vi "NI 9260 Synchronization 9775 (Host).vi"() -> ()   [LabVIEW 2021]
uses:
  <vilib>/LabVIEW Targets/FPGA/cRIO/shared/nicrio_ModuleControls/nicrio_cRIO-9260_DataRatesRing2.ctl
  <vilib>/LabVIEW Targets/FPGA/cRIO/shared/nicrio_ModuleControls/nicrio_cRIO-9775_RecordDataRates4ChansRing.ctl
  <vilib>/FPGAPlugInAG/cRIO-9053/niLvFpga_Open_cRIO-9053.vi
  <vilib>/rvi/interface/common/dynamic/niFpgaDynamicAddResources.vi
  <vilib>/Utility/error.llb/Error Cluster From Error Code.vi
  <vilib>/rvi/errors/niLvFpgaAdjustHostInterfaceError.vi
  <vilib>/rvi/interface/common/niFpgaWaitOnOcc.vi
  <vilib>/FPGAPlugInAG/Dynamic/niLvFpga_Run_Dynamic.vi
  <vilib>/FPGAPlugInAG/Dynamic/niLvFpga_Close_Dynamic.vi
  <vilib>/rvi/interface/nirviOpenFPGA/nirviOpenFPGA.xnode
  FPGA Bitfiles/crio-ni9260_FPGATarget_NI9260Synchroniz_lbmddMo-IB0.lvbitx
  NI 9260 Synchronization 9775 (FPGA).vi
  <vilib>/rvi/interface/nirviReadWriteControl/nirviReadWriteControl.xnode
  <vilib>/rvi/interface/nirviMethod/nirviMethod.xnode
  <vilib>/rvi/interface/nirviCloseFPGA/nirviCloseFPGA.xnode
  <vilib>/rvi/interface/Simulation/niFpgaSimulationCallBeginRW.vi
  <vilib>/FPGAPlugInAG/Dynamic/niLvFpga_WriteFifo_Dynamic.vi
  <vilib>/rvi/errors/niLvFpgaMergeErrorWithErrorCode.vi
  <vilib>/FPGAPlugInAG/Dynamic/niLvFpga_ConfigureFifo_Dynamic.vi
  <vilib>/Analysis/NI_AALPro.lvlib
  NiFpgaLv.dll
  <vilib>/FPGAPlugInAG/Dynamic/niLvFpga_ReadFifo_Dynamic.vi
panel:
  in  "NI9775 Data Rate":T1=1 items=["20.000 MS/s (NI 9775)"=1, "10.00 MS/s (NI 9775)"=2, "6.667 MS/s (NI 9775)"=3, "5.000 MS/s (NI 9775)"=4, "2.500 MS/s (NI 9775)"=8, "1.667 MS/s (NI 9775)"=12, "1.250 MS/s (NI 9775)"=16, "1.000 MS/s (NI 9775)"=20, "833.333 KS/s (NI 9775)"=24, "714.286 KS/s (NI 9775)"=28, "625.000 KS/s (NI 9775)"=32, "555.556 KS/s (NI 9775)"=36, "500.000 KS/s (NI 9775)"=40, "454.545 KS/s (NI 9775)"=44, "416.667 KS/s (NI 9775)"=48, "384.615 KS/s (NI 9775)"=52, "357.143 KS/s (NI 9775)"=56, "333.333 KS/s (NI 9775)"=60, "312.500 KS/s (NI 9775)"=64, "294.118 KS/s (NI 9775)"=68, "277.778 KS/s (NI 9775)"=72, "263.158 KS/s (NI 9775)"=76, "250.000 KS/s (NI 9775)"=80, "238.095 KS/s (NI 9775)"=84, "227.273 KS/s (NI 9775)"=88, "217.391 KS/s (NI 9775)"=92, "208.333 KS/s (NI 9775)"=96, "200.000 KS/s (NI 9775)"=100, "192.308 KS/s (NI 9775)"=104, "185.185 KS/s (NI 9775)"=108, "178.571 KS/s (NI 9775)"=112, "172.414 KS/s (NI 9775)"=116, "166.667 KS/s (NI 9775)"=120, "161.290 KS/s (NI 9775)"=124, "156.250 KS/s (NI 9775)"=128, "151.515 KS/s (NI 9775)"=132, "147.059 KS/s (NI 9775)"=136, "142.857 KS/s (NI 9775)"=140, "138.889 KS/s (NI 9775)"=144, "135.135 KS/s (NI 9775)"=148, "131.579 KS/s (NI 9775)"=152, "128.205 KS/s (NI 9775)"=156, "125.000 KS/s (NI 9775)"=160, "121.951 KS/s (NI 9775)"=164, "119.048 KS/s (NI 9775)"=168, "116.279 KS/s (NI 9775)"=172, "113.636 KS/s (NI 9775)"=176, "111.111 KS/s (NI 9775)"=180, "108.696 KS/s (NI 9775)"=184, "106.383 KS/s (NI 9775)"=188, "104.167 KS/s (NI 9775)"=192, "102.041 KS/s (NI 9775)"=196, "100.000 KS/s (NI 9775)"=200, "50.000 KS/s (NI 9775)"=400, "33.333 KS/s (NI 9775)"=600, "25.000 KS/s (NI 9775)"=800, "20.000 KS/s (NI 9775)"=1000, "16.667 KS/s (NI 9775)"=1200, "14.286 KS/s (NI 9775)"=1400, "12.500 KS/s (NI 9775)"=1600, "11.111 KS/s (NI 9775)"=1800, "10.000 KS/s (NI 9775)"=2000, "9.091 KS/s (NI 9775)"=2200, "8.333 KS/s (NI 9775)"=2400, "7.692 KS/s (NI 9775)"=2600, "7.143 KS/s (NI 9775)"=2800, "6.667 KS/s (NI 9775)"=3000, "6.250 KS/s (NI 9775)"=3200, "5.882 KS/s (NI 9775)"=3400, "5.556 KS/s (NI 9775)"=3600, "5.000 KS/s (NI 9775)"=4000, "4.762 KS/s (NI 9775)"=4200, "4.545 KS/s (NI 9775)"=4400, "4.348 KS/s (NI 9775)"=4600, "4.167 KS/s (NI 9775)"=4800, "4.000 KS/s (NI 9775)"=5000, "3.846 KS/s (NI 9775)"=5200, "3.571 KS/s (NI 9775)"=5600, "3.333 KS/s (NI 9775)"=6000, "3.125 KS/s (NI 9775)"=6400, "2.941 KS/s (NI 9775)"=6800, "2.778 KS/s (NI 9775)"=7200, "2.632 KS/s (NI 9775)"=7600, "2.500 KS/s (NI 9775)"=8000, "2.381 KS/s (NI 9775)"=8400, "2.273 KS/s (NI 9775)"=8800, "2.174 KS/s (NI 9775)"=9200, "2.083 KS/s (NI 9775)"=9600, "2.000 KS/s (NI 9775)"=10000, "1.923 KS/s (NI 9775)"=10400, "1.852 KS/s (NI 9775)"=10800, "1.786 KS/s (NI 9775)"=11200, "1.724 KS/s (NI 9775)"=11600, "1.667 KS/s (NI 9775)"=12000, "1.613 KS/s (NI 9775)"=12400, "1.563 KS/s (NI 9775)"=12800, "1.515 KS/s (NI 9775)"=13200, "1.471 KS/s (NI 9775)"=13600, "1.429 KS/s (NI 9775)"=14000, "1.389 KS/s (NI 9775)"=14400, "1.351 KS/s (NI 9775)"=14800, "1.316 KS/s (NI 9775)"=15200, "1.282 KS/s (NI 9775)"=15600, "1.250 KS/s (NI 9775)"=16000, "1.220 KS/s (NI 9775)"=16400, "1.190 KS/s (NI 9775)"=16800, "1.163 KS/s (NI 9775)"=17200, "1.136 KS/s (NI 9775)"=17600, "1.111 KS/s (NI 9775)"=18000, "1.087 KS/s (NI 9775)"=18400, "1.064 KS/s (NI 9775)"=18800, "1.042 KS/s (NI 9775)"=19200, "1.020 KS/s (NI 9775)"=19600, "1.000 KS/s (NI 9775)"=20000, "0.980 KS/s (NI 9775)"=20400, "0.962 KS/s (NI 9775)"=20800, "0.943 KS/s (NI 9775)"=21200, "0.926 KS/s (NI 9775)"=21600, "0.909 KS/s (NI 9775)"=22000, "0.893 KS/s (NI 9775)"=22400, "0.877 KS/s (NI 9775)"=22800, "0.862 KS/s (NI 9775)"=23200, "0.847 KS/s (NI 9775)"=23600, "0.833 KS/s (NI 9775)"=24000, "0.820 KS/s (NI 9775)"=24400, "0.806 KS/s (NI 9775)"=24800, "0.794 KS/s (NI 9775)"=25200, "0.781 KS/s (NI 9775)"=25600, "0.694 KS/s (NI 9775)"=28800, "0.625 KS/s (NI 9775)"=32000, "0.568 KS/s (NI 9775)"=35200, "0.521 KS/s (NI 9775)"=38400, "0.446 KS/s (NI 9775)"=44800, "0.391 KS/s (NI 9775)"=51200, "0.347 KS/s (NI 9775)"=57600, "0.313 KS/s (NI 9775)"=64000]
  out "host rate (ms)":u32
  out "Analog Input 2":waveform(dbl)(graph)
  in  "Waveform":T2(ring)=enum."Sine Wave"
  in  "NI 9260 Data Rate":T3=1 items=["51.200 kS/s (NI 9260)"=1, "25.600 kS/s (NI 9260)"=2, "17.067 kS/s (NI 9260)"=3, "12.800 kS/s (NI 9260)"=4, "10.240 kS/s (NI 9260)"=5, "8.533 kS/s (NI 9260)"=6, "7.314 kS/s (NI 9260)"=7, "6.400 kS/s (NI 9260)"=8, "5.689 kS/s (NI 9260)"=9, "5.120 kS/s (NI 9260)"=10, "4.654 kS/s (NI 9260)"=11, "4.267 kS/s (NI 9260)"=12, "3.938 kS/s (NI 9260)"=13, "3.657 kS/s (NI 9260)"=14, "3.413 kS/s (NI 9260)"=15, "3.200 kS/s (NI 9260)"=16, "3.012 kS/s (NI 9260)"=17, "2.845 kS/s (NI 9260)"=18, "2.695 kS/s (NI 9260)"=19, "2.560 kS/s (NI 9260)"=20, "2.438 kS/s (NI 9260)"=21, "2.328 kS/s (NI 9260)"=22, "2.226 kS/s (NI 9260)"=23, "2.133 kS/s (NI 9260)"=24, "2.048 kS/s (NI 9260)"=25, "1.969 kS/s (NI 9260)"=26, "1.896 kS/s (NI 9260)"=27, "1.829 kS/s (NI 9260)"=28, "1.765 kS/s (NI 9260)"=29, "1.707 kS/s (NI 9260)"=30, "1.652 kS/s (NI 9260)"=31]
  out "Analog Input":waveform(dbl)[](graph)
  out "NI 9230 FIFO Time Out":bool
  in  "Host Loop Rate (ms)":u32=100
  out "NI 9260 FIFO Time Out":bool
  in  "Waveform Settings":T4(array[cluster])=[{"Frequency (Hz)"=100.0, "Amplitude (V)"=3.0, "Offset (V)"=0.0, "Phase (deg)"=0.0}, {"Frequency (Hz)"=100.0, "Amplitude (V)"=3.0, "Offset (V)"=0.0, "Phase (deg)"=0.0}]
  in  "stop":bool
  out "FPGA Error out":errorcluster
  in  "Number of Samples per channel":dbl=2048.0 format="%.4p"
  out "Analog Output":waveform(dbl)[](graph)
  out "Host Error out":errorcluster
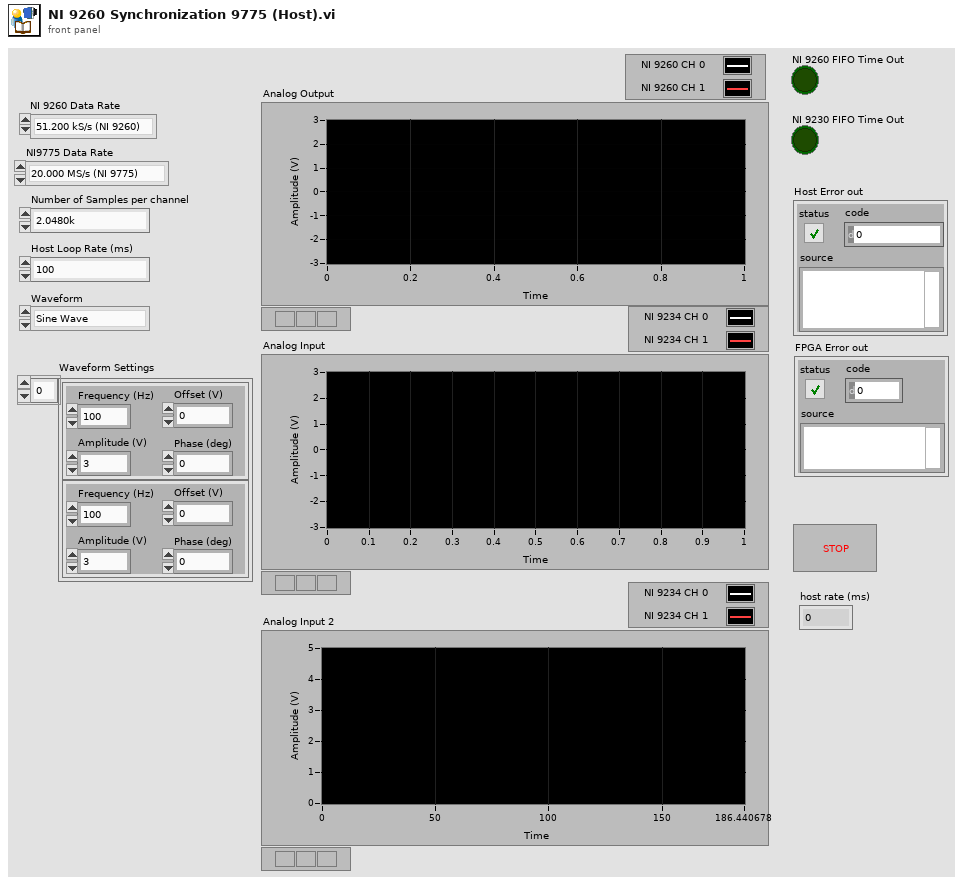
[diagram p1: front panel]
types:
  T1 = typedef "nicrio_cRIO-9775_RecordDataRates4ChansRing.ctl" = u16
  T2 = enum16{"Sawtooth Wave", "Square Wave", "Sine Wave"}
  T3 = typedef "nicrio_cRIO-9260_DataRatesRing2.ctl" = u8
  T4 = cluster{"Frequency (Hz)":dbl, "Amplitude (V)":dbl, "Offset (V)":dbl, "Phase (deg)":dbl}[]
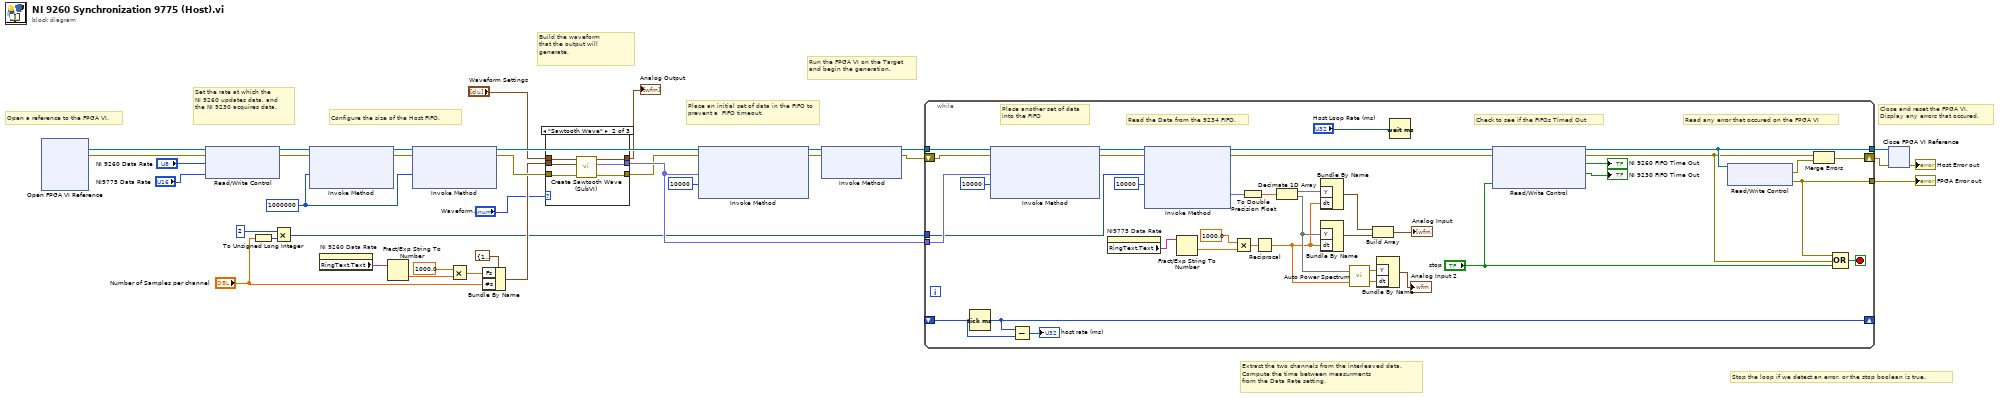
[diagram p0: block diagram]
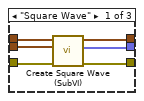
[diagram p2: hidden frame]
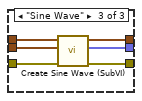
[diagram p3: hidden frame]
diagram:
  w2 = u32 1000000 ("Requested Depth")
  # "Build the waveform \nthat the output will generate."
  # "Extract the two channels from the interleaved data.\nCompute the time between measurments \nfrom the Data Rate setting."
  # "Place an initial set of data in the FIFO to prevent a  FIFO timeout."
  # "Stop the loop if we detect an error, or the stop boolean is true."
  # "Configure the size of the Host FIFO."
  # "Set the rate at which the \nNI 9260 updates data, and\nthe NI 9230 acquires data."
  # "Close and reset the FPGA VI. \nDisplay any errors that occured."
  # "Run the FPGA VI on the Target and begin the generation."
  # "Open a reference to the FPGA VI."
  n1 = xnode "Open FPGA VI Reference"() -> ("FPGA VI Reference Out"=w33:refnum<k20>, "error out"=w35:errorcluster)  [unwired: 2 in]
  n2 = xnode "Read/Write Control"("FPGA VI Reference In"=w33, "error in"=w35, "NI 9260 Data Rate"="NI 9260 Data Rate", "NI9775 Data Rate"="NI9775 Data Rate") -> ("FPGA VI Reference Out"=w15:refnum<k20>, "error out"=w23:errorcluster)
  n3 = To Unsigned Long Integer(number="Number of Samples per channel") -> (unsigned 32bit integer=w28:u32)
  n4 = Multiply(x=u32 2, y=w28) -> (x*y=w3:u32)
  n5 = xnode "Invoke Method"("FPGA VI Reference In"=w15, "error in"=w23, "Requested Depth"=w2) -> ("FPGA VI Reference Out"=w14:refnum<k20>, "error out"=w16:errorcluster)  [unwired: 1 out]
  n6 = property on="NI 9260 Data Rate" class="Ring (strict)"() -> ("RingText.Text"=w5:string)  [unwired: 2 in, 2 out]
  n7 = Fract/Exp String To Number(string=w5) -> (number=w31:dbl)  [unwired: 3 in, 1 out]
  n8 = xnode "Invoke Method"("FPGA VI Reference In"=w14, "error in"=w16, "Requested Depth"=w2) -> ("FPGA VI Reference Out"=w25:refnum<k20>, "error out"=w13:errorcluster)  [unwired: 1 out]
  n9 = Multiply(x=1000.0, y=w31) -> (x*y=w20:dbl)
  n10 = Bundle By Name(cluster=cluster{"Fs":dbl, "#s":dbl} {"Fs"=1000.0, "#s"=1000.0} ("sampling info"), "Fs"=w20, "#s"="Number of Samples per channel") -> (w11:cluster{"Fs":dbl, "#s":dbl})
  n11 = case shown="\"Sawtooth Wave\"" "Waveform" {
    tunnel: w13 -> [w39 w45 w53]
    tunnel: "Waveform Settings" -> [w41 w47 w52]
    tunnel: w11 -> [w40 w46 w51]
    tunnel: [w36 w42 w50] -> w10
    tunnel: [w38 w43 w49] -> w9
    tunnel: [w37 w44 w48] -> w7
    frame "Square Wave" {
      n12 = call "Create Square Wave (SubVI).vi"("error in (no error)"=w39, "sampling info"=w40, "Sine Waveform Settings"=w41) -> ("error out"=w38:errorcluster, "FXP Sinewave"=w36:fxp<+/-,24,4>[], "Voltage Output Waveform"=w37:waveform(dbl)[])  [unwired: 6 in]
    }
    frame "Sawtooth Wave" {
      n13 = call "Create Sawtooth Wave (SubVI).vi"("error in (no error)"=w45, "sampling info"=w46, "Sine Waveform Settings"=w47) -> ("error out"=w43:errorcluster, "FXP Sinewave"=w42:fxp<+/-,24,4>[], "Voltage Output Waveform"=w44:waveform(dbl)[])  [unwired: 6 in]
    }
    frame "Sine Wave" {
      n14 = call "Create Sine Wave (SubVI).vi"("error in (no error)"=w53, "sampling info"=w51, "Sine Waveform Settings"=w52) -> ("error out"=w49:errorcluster, "FXP Sinewave"=w50:fxp<+/-,24,4>[], "Voltage Output Waveform"=w48:waveform(dbl)[])  [unwired: 6 in]
    }
  }
  "Analog Output" <- w7
  n15 = xnode "Invoke Method"("FPGA VI Reference In"=w25, "error in"=w9, "Data"=w10, "Timeout (ms)"=10000) -> ("FPGA VI Reference Out"=w24:refnum<k20>, "error out"=w26:errorcluster)  [unwired: 1 out]
  n16 = xnode "Invoke Method"("FPGA VI Reference In"=w24, "error in"=w26) -> ("FPGA VI Reference Out"=w27:refnum<k20>, "error out"=w8:errorcluster)  [unwired: 1 in]
  n17 = while {
    tunnel: w27 -> [w91]
    tunnel: w10 -> [w90]
    tunnel: [w80] -> w21
    tunnel: [w86] -> w17
    shift-right: [w68] -> w30
    shift-left: w8 -> [w66]
    shift-right: [w58] -> _
    shift-left: _ -> [w57]
    tunnel: w3 -> [w55]
    stop <- w88 stop-if-true
    # "Check to see if the FIFOs Timed Out"
    # "Read any error that occured on the FPGA VI"
    # "Read the Data from the 9234 FIFO."
    # "Place another set of data\ninto the FIFO"
    n18 = Tick Count (ms)() -> (millisecond timer value=w58:u32)
    n19 = xnode "Invoke Method"("FPGA VI Reference In"=w91, "error in"=w66, "Data"=w90, "Timeout (ms)"=10000) -> ("FPGA VI Reference Out"=w85:refnum<k20>, "error out"=w84:errorcluster)  [unwired: 1 out]
    n20 = Subtract(x=w58, y=w57) -> (x-y=→"host rate (ms)":u32)
    n21 = property on="NI9775 Data Rate" class="Ring (strict)"() -> ("RingText.Text"=w54:string)  [unwired: 2 in, 2 out]
    n22 = xnode "Invoke Method"("FPGA VI Reference In"=w85, "error in"=w84, "Number of Elements"=w55, "Timeout (ms)"=10000) -> ("FPGA VI Reference Out"=w82:refnum<k20>, "error out"=w81:errorcluster, "Data"=w79:fxp<+/-,24,7>[])  [unwired: 1 out]
    n23 = Fract/Exp String To Number(string=w54) -> (number=w76:dbl)  [unwired: 4 out]
    n24 = Multiply(x=1000.0, y=w76) -> (x*y=w77:dbl)
    n25 = To Double Precision Float(number=w79) -> (double precision float=w69:dbl[])
    n26 = Reciprocal(x=w77) -> (1/x=w62:dbl)
    n27 = Decimate 1D Array(w69) -> (w73:dbl[], w63:dbl[])
    n28 = Bundle By Name("Y"=w73, "dt"=w62) -> (w75:waveform(dbl))  [unwired: 1 out]
    n29 = Bundle By Name("Y"=w63, "dt"=w62) -> (w74:waveform(dbl))  [unwired: 1 out]
    n30 = call <vilib>:"Auto Power Spectrum.vi"("dt"=w62, "Signal (V)"=w63) -> ("df"=w60:dbl, "Power Spectrum (V^2 rms)"=w61:dbl[])
    n31 = Build Array(w75, w74) -> (→"Analog Input":waveform(dbl)[])
    n32 = Bundle By Name("Y"=w61, "dt"=w60) -> (→"Analog Input 2":waveform(dbl))  [unwired: 1 out]
    n33 = Wait (ms)(milliseconds to wait="Host Loop Rate (ms)") -> ()  [unwired: 1 out]
    n34 = xnode "Read/Write Control"("FPGA VI Reference In"=w82, "error in"=w81, "stop"="stop") -> ("FPGA VI Reference Out"=w80:refnum<k20>, "error out"=w67:errorcluster, "NI 9260 FIFO Time Out"=→"NI 9260 FIFO Time Out":bool, "NI 9230 FIFO Time Out"=→"NI 9230 FIFO Time Out":bool)
    n35 = xnode "Read/Write Control"("FPGA VI Reference In"=w80) -> ("error out"=w65:errorcluster, "FPGA Error out"=w86:errorcluster)  [unwired: 1 in, 1 out]
    n36 = Merge Errors(w67, w65) -> (w68:errorcluster)
    n37 = Compound Arithmetic op=OR(w86, w67, "stop") -> (w88:bool)
  }
  "FPGA Error out" <- w17
  n38 = xnode "Close FPGA VI Reference"("FPGA VI Reference In"=w21, "error in"=w30) -> ("error out"=→"Host Error out":errorcluster)
